vi "SW Trigger.vi"(8 "error in (no error)":errorcluster, 10 "Params":variant, 11 "SMU in":refnum<class "NI SMU.lvclass">) -> (0 "error out":errorcluster, 3 "SMU out":refnum<class "NI SMU.lvclass">)   [LabVIEW 2020, in "NI SMU.lvlib" / "NI SMU.lvclass"]
uses:
  NI SMU.lvclass
  NI SMU.lvclass/NI SMU.ctl
  <instrlib>/niDCPower/nidcpower.llb/niDCPower Send Software Edge Trigger - Signal.ctl
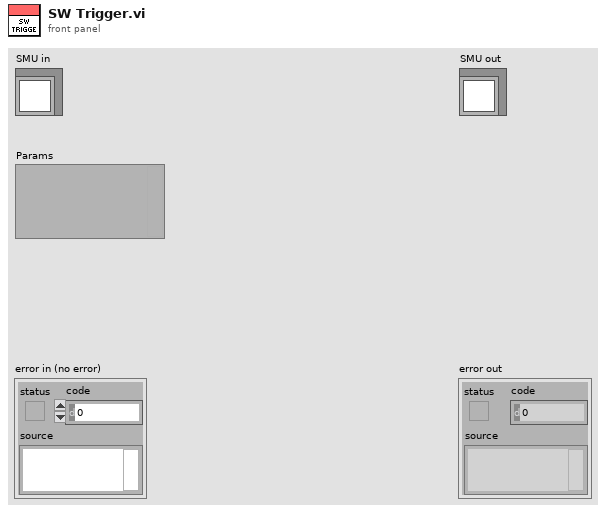
[diagram p1: front panel]
types:
  T1 = typedef "niDCPower Send Software Edge Trigger - Signal.ctl" = i32
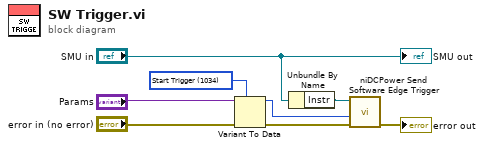
[diagram p0: block diagram]
diagram:
  w3 = T1 1034 items=["Start Trigger"=1034, "Source Trigger"=1035, "Measure Trigger"=1036, "Sequence Advance Trigger"=1037, "Pulse Trigger"=1053] ("signal")
  n1 = Variant To Data(error in="error in (no error)", type=w3, Variant="Params") -> (data=w2:T1, error out=w4:errorcluster)
  n2 = Unbundle By Name("SMU in") -> ("Instr"=w7:refnum<k15>)
  n3 = call <instrlib>:"niDCPower Send Software Edge Trigger.vi"("error in (no error)"=w4, "signal"=w2, "instrument handle"=w7) -> ("error out"=→"error out":errorcluster)  [unwired: 7 in, 1 out]
  "SMU out" <- "SMU in"
